vi "Custom_XNOR.vi"(9 "INPUT B":bool, 11 "INPUT A":bool) -> (3 "Boolean 3":bool)   [LabVIEW 2026]
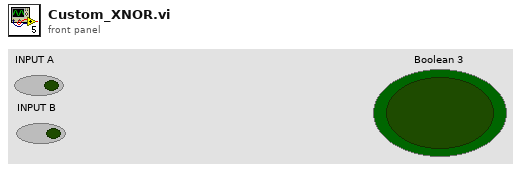
[diagram p1: front panel]
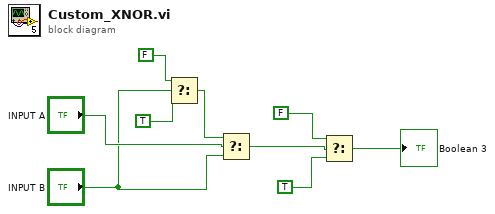
[diagram p0: block diagram]
diagram:
  n1 = Select(t=FALSE, s="INPUT B", f=TRUE) -> (s? t:f=w5:bool)
  n2 = Select(t=w5, s="INPUT A", f="INPUT B") -> (s? t:f=w2:bool)
  n3 = Select(t=FALSE, s=w2, f=TRUE) -> (s? t:f=→"Boolean 3":bool)
